vi "compare.parse.field.results.vi"(10 "Test Case #1 - Sequenced Unit Header - Hdr Length":T1={"buffer.length"=0, "start.idx"=0, "buffer"=[0, 0, 0, 0, 0, 0, 0, 0, 0], "U8"=FALSE, "exp.u8"=0, "U16"=FALSE, "exp.u16"=0, "U32"=FALSE, "exp.u32"=0, "U64"=FALSE, "exp.u64"=0} {"exp.u64" format="%.0x"; "exp.u32" format="%.0x"; "exp.u16" format="%.0x"; "exp.u8" format="%.0x"; "buffer" format="%.0x"}, 11 "Val.in":u64) -> (3 "Equal?":bool)   [LabVIEW 2020]
uses:
  parse.field.test.case.ctl
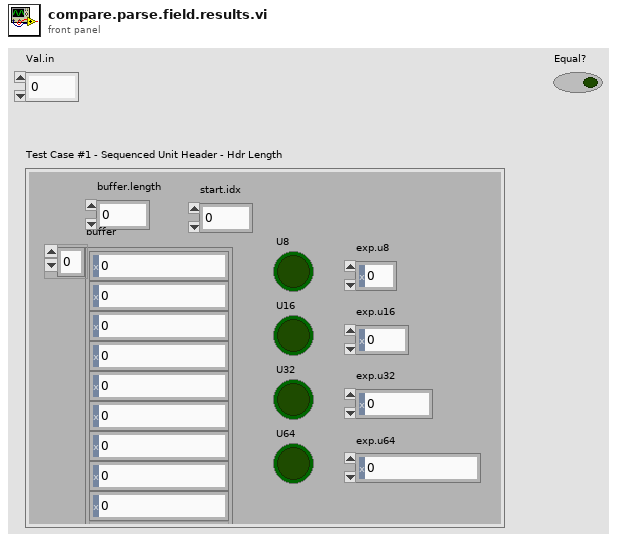
[diagram p1: front panel]
types:
  T1 = typedef "parse.field.test.case.ctl" = cluster{"buffer.length":u8, "start.idx":u8, "buffer":u64[], "U8":bool, "exp.u8":u8, "U16":bool, "exp.u16":u16, "U32":bool, "exp.u32":u32, "U64":bool, "exp.u64":u64}
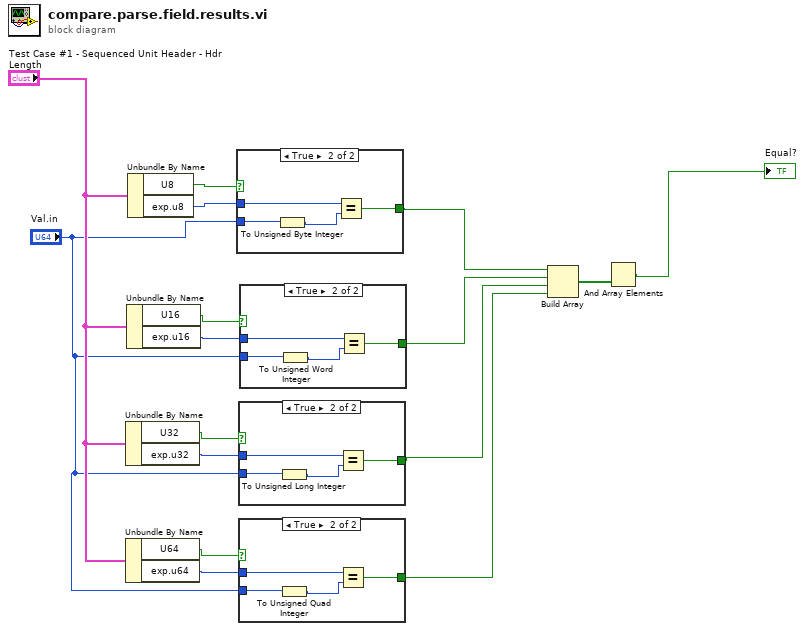
[diagram p0: block diagram]
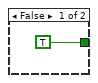
[diagram p2: hidden frame]
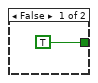
[diagram p3: hidden frame]
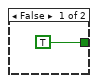
[diagram p4: hidden frame]
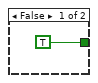
[diagram p5: hidden frame]
diagram:
  n1 = Unbundle By Name("Test Case #1 - Sequenced Unit Header - Hdr Length") -> ("U32"=w8:bool, "exp.u32"=w7:u32)
  n2 = Unbundle By Name("Test Case #1 - Sequenced Unit Header - Hdr Length") -> ("U64"=w6:bool, "exp.u64"=w5:u64)
  n3 = Unbundle By Name("Test Case #1 - Sequenced Unit Header - Hdr Length") -> ("U16"=w10:bool, "exp.u16"=w9:u16)
  n4 = Unbundle By Name("Test Case #1 - Sequenced Unit Header - Hdr Length") -> ("U8"=w16:bool, "exp.u8"=w15:u8)
  n5 = case shown="True" w16 {
    tunnel: "Val.in" -> [_ w21]
    tunnel: w15 -> [_ w19]
    tunnel: [TRUE w18] -> w14
    frame False {
    }
    frame True {
      n6 = To Unsigned Byte Integer(number=w21) -> (unsigned 8bit integer=w20:u8)
      n7 = Equal?(x=w19, y=w20) -> (x = y?=w18:bool)
    }
  }
  n8 = case shown="True" w8 {
    tunnel: "Val.in" -> [_ w26]
    tunnel: w7 -> [_ w24]
    tunnel: [TRUE w23] -> w2
    frame False {
    }
    frame True {
      n9 = To Unsigned Long Integer(number=w26) -> (unsigned 32bit integer=w25:u32)
      n10 = Equal?(x=w24, y=w25) -> (x = y?=w23:bool)
    }
  }
  n11 = case shown="True" w6 {
    tunnel: "Val.in" -> [_ w31]
    tunnel: w5 -> [_ w29]
    tunnel: [TRUE w28] -> w1
    frame False {
    }
    frame True {
      n12 = To Unsigned Quad Integer(1:w31) -> (0:w30:u64)
      n13 = Equal?(x=w29, y=w30) -> (x = y?=w28:bool)
    }
  }
  n14 = case shown="True" w10 {
    tunnel: "Val.in" -> [_ w36]
    tunnel: w9 -> [_ w34]
    tunnel: [TRUE w33] -> w13
    frame False {
    }
    frame True {
      n15 = To Unsigned Word Integer(number=w36) -> (unsigned 16bit integer=w35:u16)
      n16 = Equal?(x=w34, y=w35) -> (x = y?=w33:bool)
    }
  }
  n17 = Build Array(w14, w13, w2, w1) -> (w12:bool[])
  n18 = And Array Elements(Boolean array=w12) -> (logical AND=→"Equal?":bool)
